vi "ClearBuffers.vi"(8 "Error In":errorcluster, 10 "Measure Configurations":T1[](array[typedef]) {"Count" min=1 step=1}, 11 "Keithley 2602 In":refnum<visa-resource-name>) -> (0 "Error Out":errorcluster, 3 "Keithley 2602 Out":refnum<visa-resource-name>)   [LabVIEW 2012]
uses:
  MeasureConfiguration.ctl
  driver/Public/Controls/SMU.ctl
  driver/Keithley-2602.lvlib
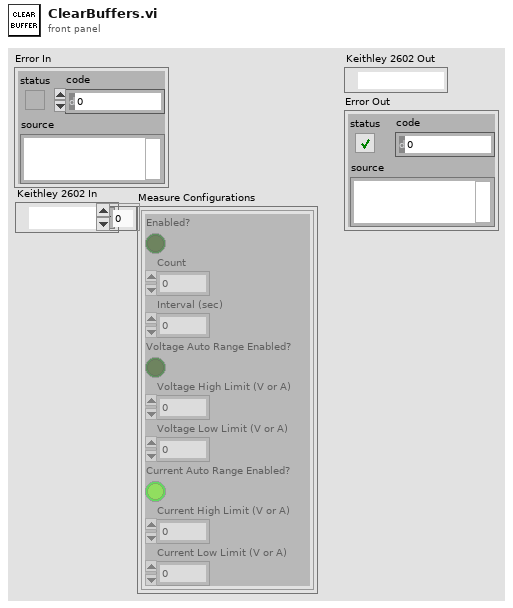
[diagram p1: front panel]
types:
  T1 = typedef "MeasureConfiguration.ctl" = cluster{"Enabled?":bool, "Count":u8, "Interval (sec)":dbl, "Voltage Auto Range Enabled?":bool, "Voltage High Limit (V or A)":dbl, "Voltage Low Limit (V or A)":dbl, "Current Auto Range Enabled?":bool, "Current High Limit (V or A)":dbl, "Current Low Limit (V or A)":dbl}
  T2 = typedef "Keithley-2602.lvlib/SMU.ctl" = enum16{"A", "B"}
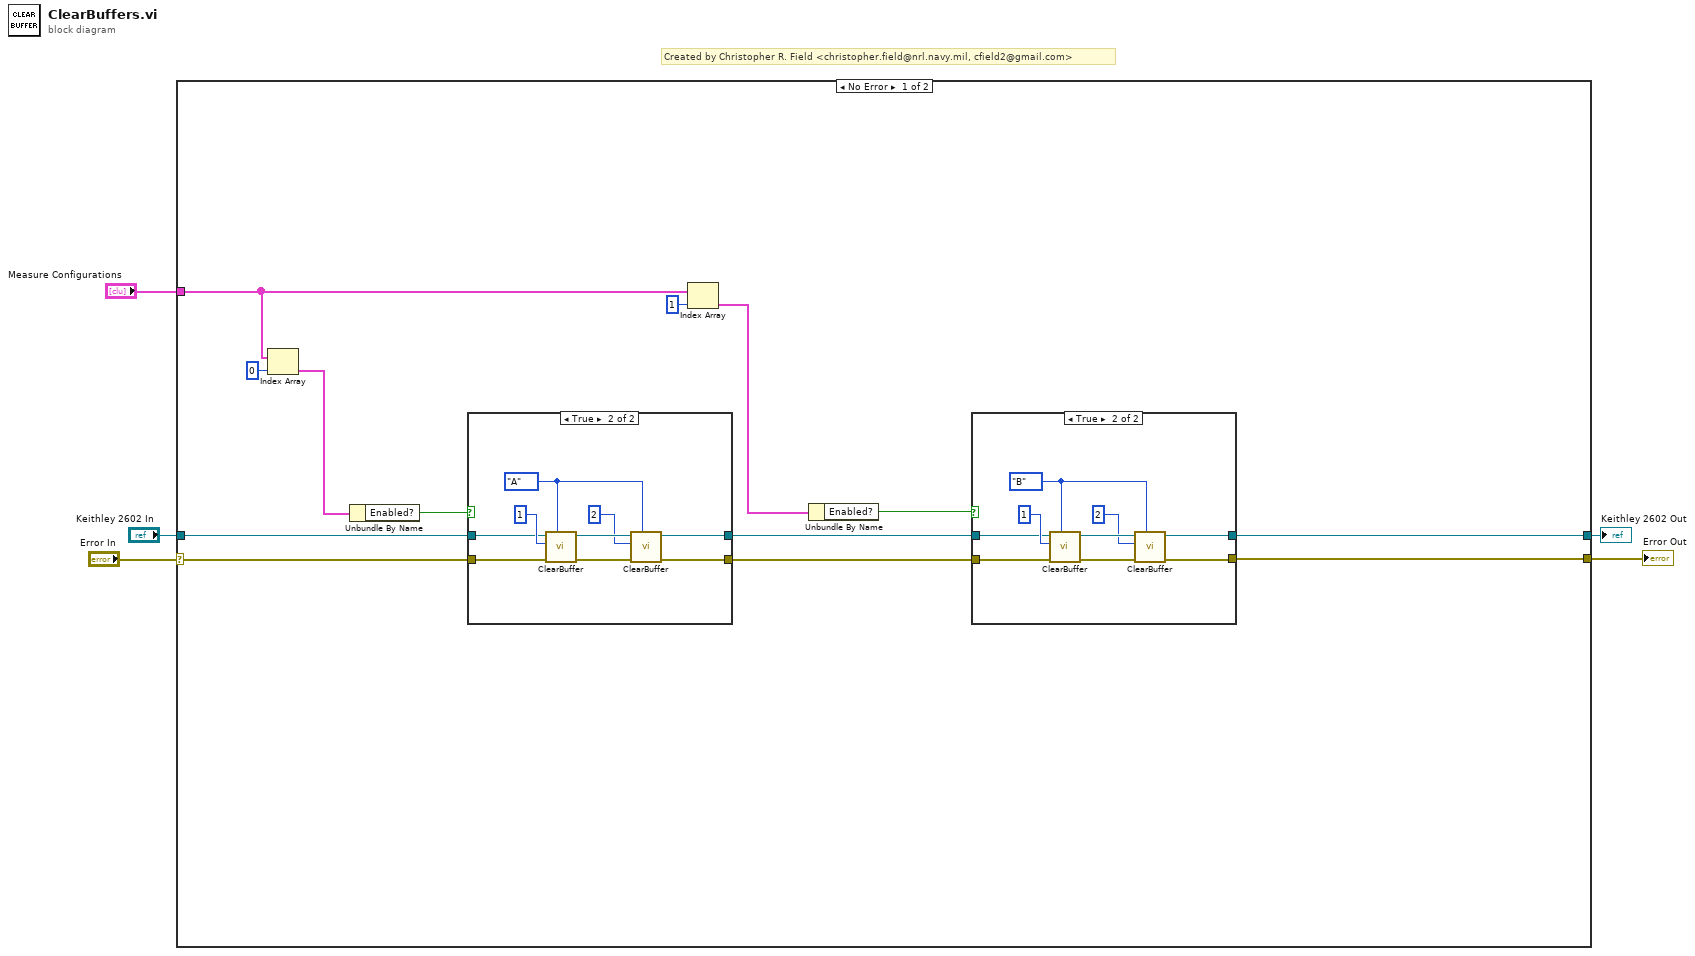
[diagram p0: block diagram]
diagram:
  # "Created by Christopher R. Field <christopher.field@nrl.navy.mil, cfield2@gmail.com>"
  n1 = case shown="No Error" "Error In" {
    selector: "Error In" -> [w18 w41]
    tunnel: "Keithley 2602 In" -> [w17 w42]
    tunnel: [w14 w41] -> w2
    tunnel: [w13 w42] -> w3
    tunnel: "Measure Configurations" -> [w8 _]
    frame No Error {
      n2 = Index Array(array=w8, index=0) -> (element=w7:T1)
      n3 = Unbundle By Name(w7) -> ("Enabled?"=w6:bool)
      n4 = case shown="True" w6 {
        tunnel: w18 -> [w30 w37]
        tunnel: w17 -> [w31 w36]
        tunnel: [w31 w33] -> w15
        tunnel: [w30 w32] -> w16
        frame False {
        }
        frame True {
          w35 = SMU."A" ("SMU")
          n5 = call "ClearBuffer.vi"("SMU"=w35, "Error In"=w37, "Buffer"=u8 1, "Keithley 2602 In"=w36) -> ("Error Out"=w38:errorcluster, "Keithley 2602 Out"=w40:refnum<visa-resource-name>)  [unwired: 6 in]
          n6 = call "ClearBuffer.vi"("SMU"=w35, "Error In"=w38, "Buffer"=u8 2, "Keithley 2602 In"=w40) -> ("Error Out"=w32:errorcluster, "Keithley 2602 Out"=w33:refnum<visa-resource-name>)  [unwired: 6 in]
        }
      }
      n7 = Index Array(array=w8, index=1) -> (element=w11:T1)
      n8 = Unbundle By Name(w11) -> ("Enabled?"=w10:bool)
      n9 = case shown="True" w10 {
        tunnel: w16 -> [w19 w26]
        tunnel: w15 -> [w20 w25]
        tunnel: [w20 w22] -> w13
        tunnel: [w19 w21] -> w14
        frame False {
        }
        frame True {
          w24 = SMU."B" ("SMU")
          n10 = call "ClearBuffer.vi"("SMU"=w24, "Error In"=w26, "Buffer"=u8 1, "Keithley 2602 In"=w25) -> ("Error Out"=w27:errorcluster, "Keithley 2602 Out"=w29:refnum<visa-resource-name>)  [unwired: 6 in]
          n11 = call "ClearBuffer.vi"("SMU"=w24, "Error In"=w27, "Buffer"=u8 2, "Keithley 2602 In"=w29) -> ("Error Out"=w21:errorcluster, "Keithley 2602 Out"=w22:refnum<visa-resource-name>)  [unwired: 6 in]
        }
      }
    }
    frame Error {
    }
  }
  "Keithley 2602 Out" <- w3
  "Error Out" <- w2
